vi "Read image data.vi"(8 "error in (no error)":errorcluster, 11 "data_loder_single_image in":refnum<class "data_loder_single_image.lvclass">) -> (0 "error out":errorcluster, 2 "image data":T1, 3 "data_loder_single_image out":refnum<class "data_loder_single_image.lvclass">)   [LabVIEW 2017, in "data_loder_single_image.lvclass"]
uses:
  data_loder_single_image.lvclass
  <vilib>/picture/picture.llb/imagedata.ctl
  data_loder_single_image.lvclass/data_loder_single_image.ctl
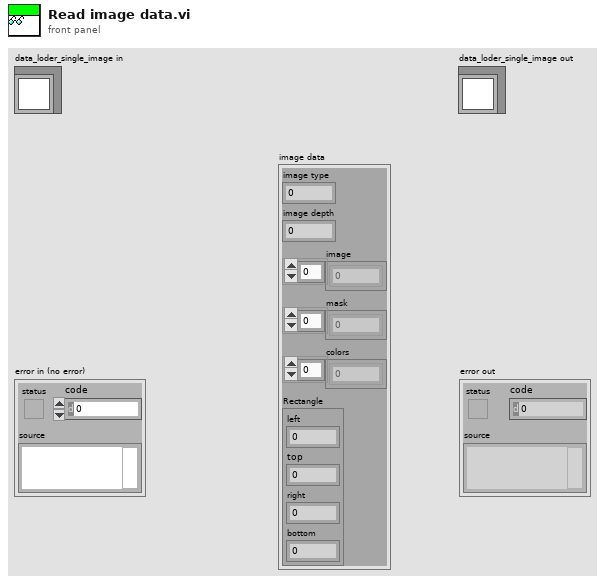
[diagram p1: front panel]
types:
  T1 = typedef "imagedata.ctl" = cluster{"image type":i32, "image depth":i32, "image":u8[], "mask":u8[], "colors":u32[], "Rectangle":cluster{"left":i16, "top":i16, "right":i16, "bottom":i16}}
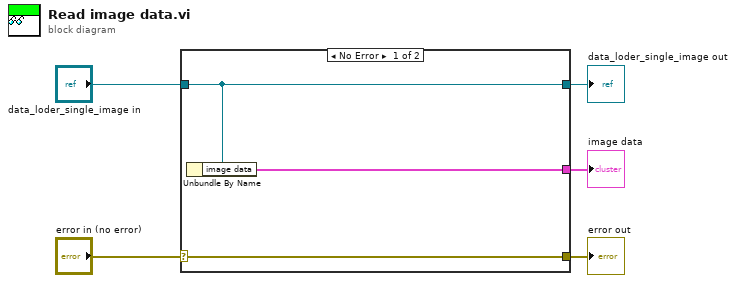
[diagram p0: block diagram]
diagram:
  n1 = case shown="No Error" "error in (no error)" {
    selector: "error in (no error)" -> [w8 w9]
    tunnel: [w8 w9] -> w4
    tunnel: [w7 w10] -> w2
    tunnel: "data_loder_single_image in" -> [w7 w10]
    tunnel: [w6 _] -> w1
    frame No Error {
      n2 = Unbundle By Name(w7) -> ("image data"=w6:T1)
    }
    frame Error {
    }
  }
  "error out" <- w4
  "data_loder_single_image out" <- w2
  "image data" <- w1
